vi "Paste Cover Section.vi"(8 "Error In":errorcluster, 9 "Mine Index (row, column)":cluster{"x":i16, "y":i16}, 10 "Pasteboard Picture":picture, 11 "Cover Picture":picture) -> (0 "Error Out":errorcluster, 3 "Output Picture":picture)   [LabVIEW 2011]
uses:
  <vilib>/picture/picture.llb/Draw True-Color Pixmap.vi
panel:
  # "="
  # "+"
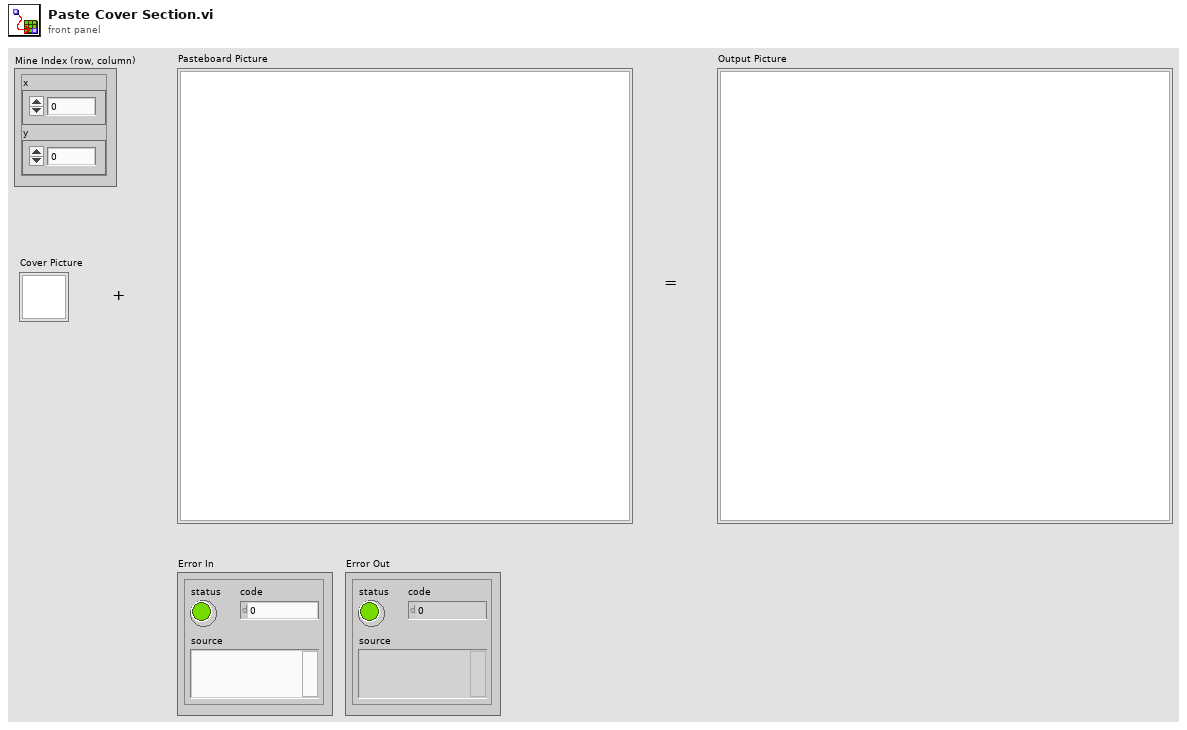
[diagram p1: front panel]
types:
  T1 = typedef "imagedata.ctl" = cluster{"image type":i32, "image depth":i32, "image":u8[], "mask":u8[], "colors":u32[], "Rectangle":cluster{"left":i16, "top":i16, "right":i16, "bottom":i16}}
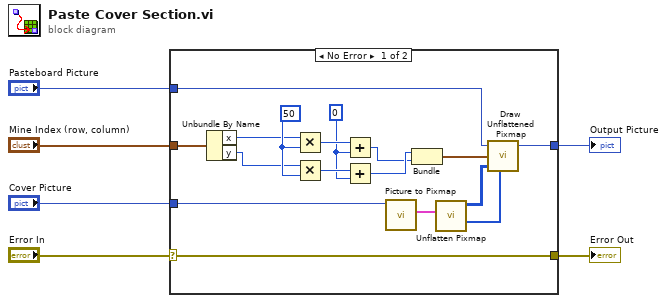
[diagram p0: block diagram]
diagram:
  n1 = case shown="No Error" "Error In" {
    selector: "Error In" -> [w7 w24]
    tunnel: "Cover Picture" -> [w16 _]
    tunnel: "Mine Index (row, column)" -> [w15 _]
    tunnel: "Pasteboard Picture" -> [w9 w25]
    tunnel: [w8 w25] -> w3
    tunnel: [w7 w24] -> w1
    frame No Error {
      w20 = i16 0
      w23 = i16 50
      n2 = Unbundle By Name(w15) -> ("x"=w14:i16, "y"=w13:i16)
      n3 = Multiply(x=w14, y=w23) -> (x*y=w22:i16)
      n4 = Multiply(x=w13, y=w23) -> (x*y=w21:i16)
      n5 = Add(x=w22, y=w20) -> (x+y=w17:i16)
      n6 = Add(x=w21, y=w20) -> (x+y=w18:i16)
      n7 = call <vilib>:"Picture to Pixmap.vi"("picture"=w16) -> ("image data"=w10:T1)  [unwired: 9 in, 1 out]
      n8 = Bundle(w18, w17) -> (w19:cluster{i16, i16})  [unwired: 1 in]
      n9 = call <vilib>:"Unflatten Pixmap.vi"("image data"=w10) -> ("24-bit pixmap"=w12:u32[][], "mask"=w11:u8[])  [unwired: 4 in, 5 out]
      n10 = call-poly <vilib>:"Draw Unflattened Pixmap.vi"("picture"=w9, "top left point(0, 0)"=w19, "data (RGB format)"=w12, "mask"=w11) -> ("new picture"=w8:picture)  [unwired: 5 in]
    }
    frame Error {
    }
  }
  "Output Picture" <- w3
  "Error Out" <- w1
